vi "Comp_INTLK_V1.vi"() -> ()   [LabVIEW 2014]
uses:
  <vilib>/Instr/_visa.llb/VISA Configure Serial Port (Serial Instr).vi
  <vilib>/Instr/_visa.llb/VISA Configure Serial Port (Instr).vi
  Applications/National Instruments/LabVIEW 2014/examples/Instrument IO/Serial/support/Serial - Settings.ctl
panel:
  out "Available Resource Descriptions":string[](array[string])
  in  "READ":bool
  in  "Serial Settings":T1={"baud rate"=9600, "data bits"=8, "parity"=enum."None", "stop bits"=10, "flow control"=0} {"flow control" items=["None"=0, "XON/XOFF"=1, "RTS/CTS"=2, "DTR/DSR"=4]; "stop bits" items=["1.0"=10, "1.5"=15, "2.0"=20]; "data bits" min=5 max=8 step=1; "baud rate" items=["75"=75, "110"=110, "134"=134, "150"=150, "300"=300, "600"=600, "1200"=1200, "1800"=1800, "2400"=2400, "4800"=4800, "7200"=7200, "9600"=9600, "14400"=14400, "19200"=19200, "28800"=28800, "38400"=38400, "56000"=56000, "57600"=57600, "115200"=115200, "128000"=128000, "230400"=230400]}
  out "bytes read":u32
  out "Response":string
  in  "delay before read (ms)":u32=500
  in  "Select  VISA Resource":refnum<visa-resource-name>="ASRL2::INSTR"
  out "find list":string[](array[string])
  in  "String":string
  in  "Select":bool
  in  "Combo Box":string(combo)
  in  "stop":bool
  out "read buffer":string
  out "Port":bool
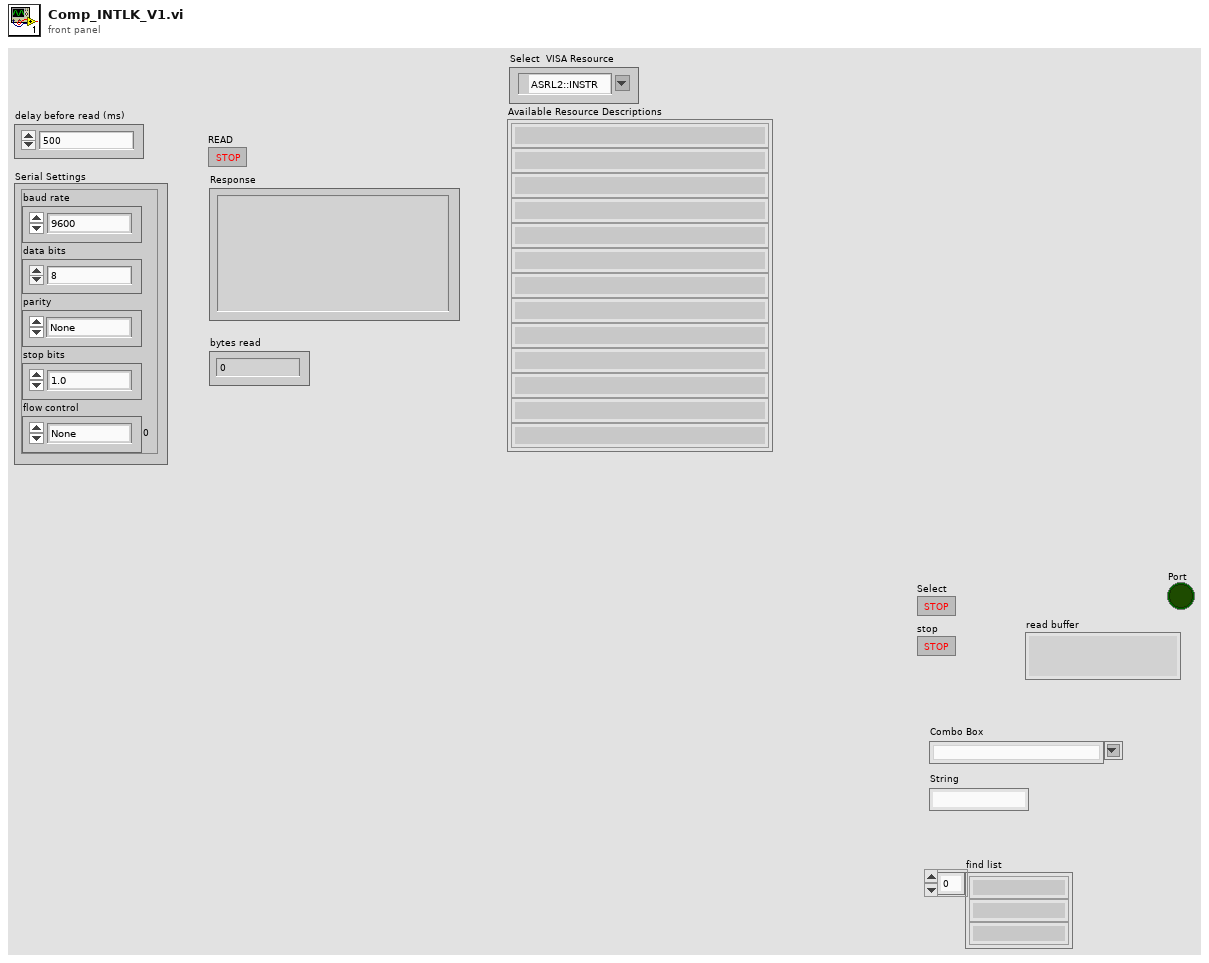
[diagram p1: front panel]
types:
  T1 = typedef "Serial - Settings.ctl" = cluster{"baud rate":u32, "data bits":u16, "parity":enum16{"None", "Odd", "Even", "Mark", "Space"}, "stop bits":u16, "flow control":u16}
  T2 = enum32{"Invalid", "Standard", "Closed", "Hidden", "Minimized", "Maximized"}
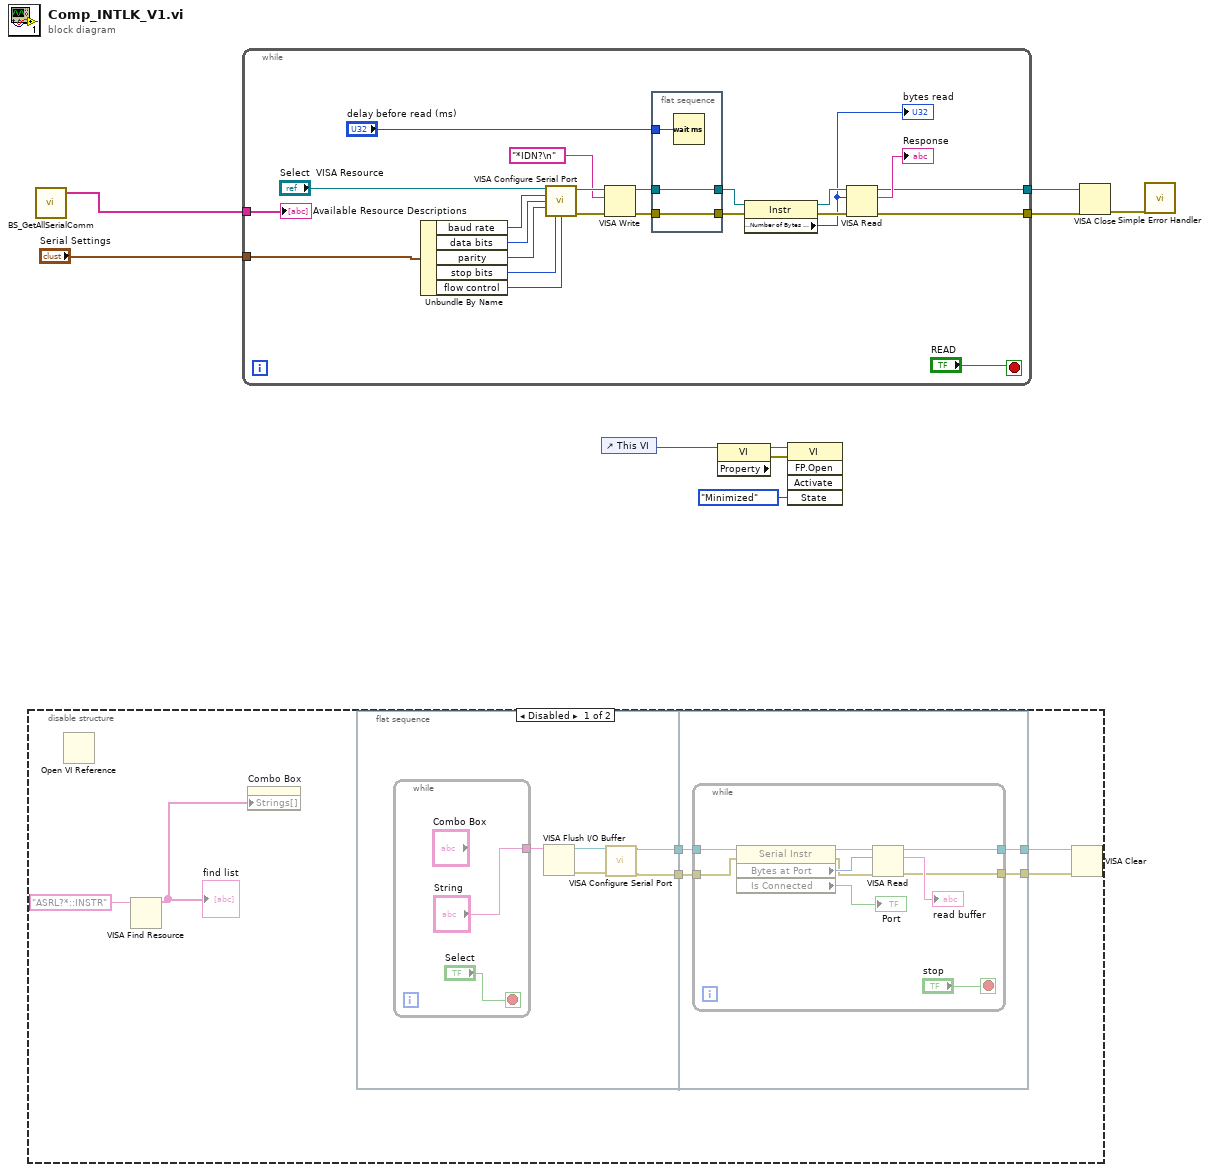
[diagram p0: block diagram]
diagram:
  n1 = disable-structure shown="Disabled" {
    frame Disabled {
      n2 = Open VI Reference() -> ()  [unwired: 6 in, 2 out]
      n3 = VISA Find Resource(11:"ASRL?*::INSTR" ("expression (\"?*\")")) -> (3:w14:string[])  [unwired: 2 in, 2 out]
      "find list" <- w14
      n4 = property on="Combo Box" class="CmbBox"("Strings[]"=w14) -> ()  [unwired: 2 in, 2 out]
      n5 = flat-sequence {
        tunnel: [w17] -> w13
        tunnel: [w18] -> w12
        tunnel: [w24] -> w10
        tunnel: [w23] -> w11
        tunnel: w13 -> [w26]
        tunnel: w12 -> [w25]
        frame #0 {
          n6 = while {
            tunnel: ["String"] -> w19
            stop <- "Select" stop-if-true
          }
          n7 = VISA Flush I/O Buffer(VISA resource name=w19) -> (VISA resource name out=w20:refnum<visa-resource-name>, error out=w16:errorcluster)  [unwired: 2 in]
          n8 = call-poly "VISA Configure Serial Port"("VISA resource name"=w20, "error in (no error)"=w16) -> ("VISA resource name out"=w17:refnum<visa-resource-name>, "error out"=w18:errorcluster)  [unwired: 12 in]
        }
        frame #1 {
          n9 = while {
            tunnel: w26 -> [w36]
            tunnel: w25 -> [w35]
            tunnel: [w30] -> w24
            tunnel: [w29] -> w23
            stop <- "stop" stop-if-true
            n10 = property class="Serial Instr"(reference=w36, error in=w35) -> (reference out=w34:refnum<visa-resource-name>, error out=w28:errorcluster, "Bytes at Port"=w33:u32, "Is Connected"=→"Port":bool)
            n11 = VISA Read(VISA resource name=w34, byte count=w33, error in (no error)=w28) -> (VISA resource name out=w30:refnum<visa-resource-name>, read buffer=→"read buffer":string, error out=w29:errorcluster)  [unwired: 1 out]
          }
        }
      }
      n12 = VISA Clear(VISA resource name=w10, error in (no error)=w11) -> ()  [unwired: 2 out]
    }
    frame Enabled {
    }
  }
  n13 = call "BS_GetAllSerialComm.vi"() -> ("names"=w8:string[])  [unwired: 2 in, 2 out]
  n14 = while {
    tunnel: "Serial Settings" -> [w47]
    tunnel: w8 -> [w40]
    tunnel: [w38] -> w6
    tunnel: [w37] -> w5
    stop <- "READ" stop-if-true
    n15 = Unbundle By Name(w47) -> ("baud rate"=w46:u32, "data bits"=w45:u16, "parity"=w44:enum16{"None", "Odd", "Even", "Mark", "Space"}, "stop bits"=w43:u16, "flow control"=w42:u16)
    n16 = call-poly "VISA Configure Serial Port"("VISA resource name"="Select  VISA Resource", "baud rate (9600)"=w46, "data bits (8)"=w45, "parity (0:none)"=w44, "stop bits (10: 1 bit)"=w43, "flow control (0:none)"=w42) -> ("VISA resource name out"=w58:refnum<visa-resource-name>, "error out"=w59:errorcluster)  [unwired: 3 in, 5 out]
    n17 = VISA Write(VISA resource name=w58, write buffer="*IDN?\n" ("Command"), error in (no error)=w59) -> (VISA resource name out=w55:refnum<visa-resource-name>, error out=w57:errorcluster)  [unwired: 1 out]
    n18 = flat-sequence {
      tunnel: w57 -> [w61]
      tunnel: [w61] -> w56
      tunnel: w55 -> [w60]
      tunnel: [w60] -> w54
      tunnel: "delay before read (ms)" -> [w62]
      frame #0 {
        n19 = Wait (ms)(milliseconds to wait=w62) -> ()  [unwired: 1 out]
      }
    }
    n20 = property class="Instr"(reference=w54, error in=w56) -> (reference out=w51:refnum<visa-resource-name>, error out=w50:errorcluster, "Serial Settings:Number of Bytes at Serial Port"=w48:u32)
    "bytes read" <- w48
    n21 = VISA Read(VISA resource name=w51, byte count=w48, error in (no error)=w50) -> (VISA resource name out=w38:refnum<visa-resource-name>, read buffer=→"Response":string, error out=w37:errorcluster)  [unwired: 1 out]
    "Available Resource Descriptions" <- w40
  }
  n22 = control-ref of="This VI"() -> (w2:refnum<vi>)
  n23 = property class="VI" props=[](reference=w2) -> (reference out=w4:refnum<vi>, error out=w3:errorcluster)  [unwired: 1 in, 1 out]
  n24 = invoke class="VI" method="FP.Open"(reference=w4, error in=w3, "State"=T2."Minimized") -> ()  [unwired: 2 in, 5 out]
  n25 = VISA Close(VISA resource name=w6, error in (no error)=w5) -> (error out=w7:errorcluster)
  n26 = call <vilib>:"Simple Error Handler.vi"("error in (no error)"=w7) -> ()  [unwired: 1 in, 8 out]
